vi "Autonomous.vi"   [LabVIEW 2017]
doc: "This VI starts when autonomous period begins, and will automatically be terminated when it ends. You can carry out timed or sensor driven operations directly to I/O or to subsystems without needing to return to the caller."
uses:
  <vilib>/Rock Robotics/WPI/SafetyOutput/WPI_SafetyOutputConfigMenu.ctl
  <vilib>/Rock Robotics/WPI/Utilities/WPI_GetSetVariantRefNum.vi
  <vilib>/Rock Robotics/Network Tables/NT Read String.vi
  <vilib>/Rock Robotics/WPI/RobotDrive/WPI_RobotDriveMecanumDrive_Cartesian.vi
types:
  T1 = typedef "WPI_JoystickDevRef.ctl" = cluster{"Device":T2}
  T2 = typedef "WPI_JoystickDeviceEnum.ctl" = enum16{"USB 0", "USB 1", "USB 2", "USB 3", "USB 4", "USB 5"}
  T3 = typedef "WPI_SafetyOutputConfigMenu.ctl" = enum16{"Enable", "Disable"}
  T4 = typedef "WPI_RobotDriveDevRef.ctl" = cluster{"DevStatus":errorcluster, "Motors[]":T5[], "Square Inputs":bool, "Max Output":dbl}
  T5 = typedef "WPI_MotorControlDeviceRef.ctl" = cluster{"DeviceStatus":errorcluster, "Type":T6, "PWM":cluster{"PWM Channel":T7, "DeadBand":T8}, "CAN":cluster{"Device Number":u8, "SetOutput VI Ref":variant, "GetOutput VI Ref":variant, "Enable VI Ref":variant, "Disable VI Ref":variant, "Data":variant}, "Invert":bool, "DIO PWM":cluster{"PWM \"Enable\" Channel":T7, "DIOChannel":T9, "PWM Rate":dbl}}
  T6 = typedef "WPI_MotorControlType.ctl" = enum16{"PWM", "CAN", "DIO PWM"}
  T7 = typedef "FPGA_DIOPWMChannel.ctl" = enum8{"PWM 0", "PWM 1", "PWM 2", "PWM 3", "PWM 4", "PWM 5", "PWM 6", "PWM 7", "PWM 8", "PWM 9", "PWM MXP 0", "PWM MXP 1", "PWM MXP 2", "PWM MXP 3", "PWM MXP 4", "PWM MXP 5", "PWM MXP 6", "PWM MXP 7", "PWM MXP 8", "PWM MXP 9", "Invalid"}
  T8 = typedef "WPI_PWMDeadband.ctl" = cluster{"Name":string, "maxPositivePwm":i32, "minPositivePwm":i32, "centerPwm":i32, "maxNegativePwm":i32, "minNegativePwm":i32, "angularRange":u16}
  T9 = typedef "FPGA_DIOChannel.ctl" = enum8{"DIO 0", "DIO 1", "DIO 2", "DIO 3", "DIO 4", "DIO 5", "DIO 6", "DIO 7", "DIO 8", "DIO 9", "DIO MXP 0", "DIO MXP 1", "DIO MXP 2", "DIO MXP 3", "DIO MXP 4", "DIO MXP 5", "DIO MXP 6", "DIO MXP 7", "DIO MXP 8", "DIO MXP 9", "DIO MXP 10", "DIO MXP 11", "DIO MXP 12", "DIO MXP 13", "DIO MXP 14", "DIO MXP 15", "SPI Port CS1", "SPI Port CS2", "SPI Port CS3", "SPI Port MISO", "SPI Port MOSI", "Invalid"}
  T10 = typedef "Command Status Info.ctl" = cluster{"Name":string, "Status":T11, "notifier out":T12}
  T11 = typedef "Completion Status.ctl" = enum16{"Successful", "Aborted", "Incomplete"}
  T12 = typedef "Completion Notifier.ctl" = refnum<notifier>
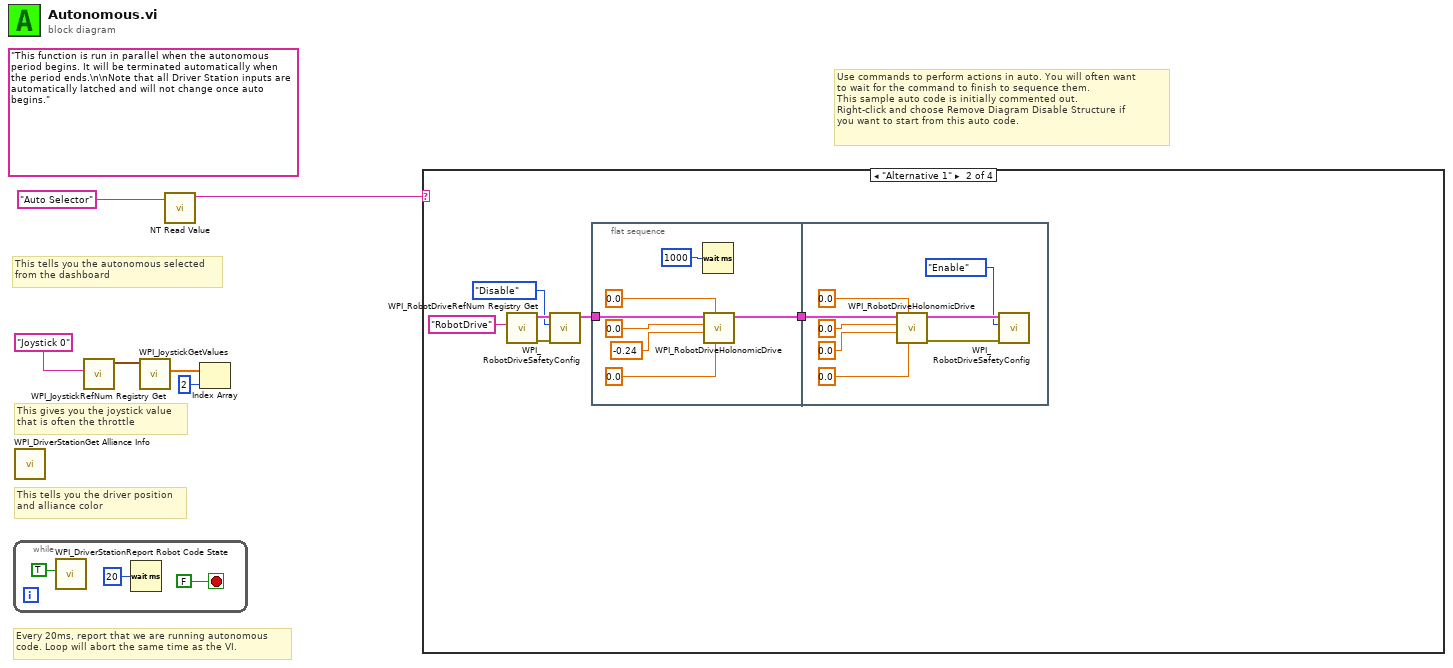
[diagram p0: block diagram]
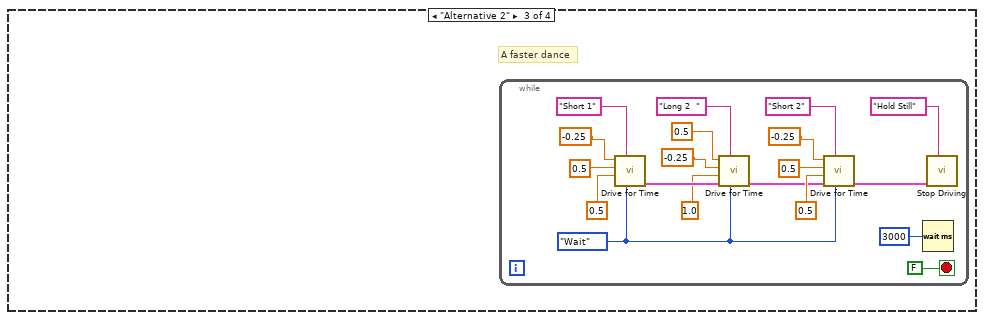
[diagram p3: hidden frame]
diagram:
  (unwired) "This function is run in parallel when the autonomous period begins. It will be terminated automatically when the period ends.\n\nNote that all Driver Station inputs are automatically latched and will not change once auto begins."
  # "This tells you the autonomous selected\nfrom the dashboard"
  # "Every 20ms, report that we are running autonomous\ncode. Loop will abort the same time as the VI."
  # "This gives you the joystick value\nthat is often the throttle"
  # "Use commands to perform actions in auto. You will often want\nto wait for the command to finish to sequence them.\nThis sample auto code is initially commented out. \nRight-click and choose Remove Diagram Disable Structure if\nyou want to start from this auto code."
  # "This tells you the driver position\nand alliance color"
  n1 = while {
    stop <- FALSE stop-if-true
    n2 = call <vilib>:"WPI_DriverStationReport Robot Code State.vi"("Autonomous"=TRUE) -> ()  [unwired: 10 in, 1 out]
    n3 = Wait (ms)(milliseconds to wait=u32 20) -> ()  [unwired: 1 out]
  }
  n4 = call <vilib>:"WPI_DriverStationGet Alliance Info.vi"() -> ()  [unwired: 12 out]
  n5 = call <vilib>:"WPI_JoystickRefNum Registry Get.vi"("refnum name"="Joystick 0") -> ("JoystickDevRef"=w5:T1)  [unwired: 1 in, 9 out]
  n6 = call <vilib>:"WPI_JoystickGetValues.vi"("JoystickDevRef"=w5) -> ("Axes"=w4:dbl[])  [unwired: 6 in, 4 out]
  n7 = call-poly <vilib>:"NT Read Value.vi"("Name"="Auto Selector") -> ("String"=w1:string)  [unwired: 9 in, 1 out]
  n8 = Index Array(array=w4, index=2) -> ()  [unwired: 1 out]
  n9 = case shown="\"Alternative 1\"" w1 {
    frame Default {
      # "You can put your main auto here, or you can right-click on the case and make any\nother frame be the default case."
      # "This is the frame that will execute if no selection is made, or if it is not recognized"
    }
    frame "Alternative 1" {
      n10 = call <vilib>:"WPI_RobotDriveRefNum Registry Get.vi"("refnum name"="RobotDrive") -> ("error out"=w13:errorcluster, "RobotDriveDevRef"=w14:T4)  [unwired: 9 in]
      n11 = call <vilib>:"WPI_RobotDriveSafetyConfig.vi"("error in (no error)"=w13, "mode"=WPI_SafetyOutputConfigMenu."Disable", "RobotDriveDevRef"=w14) -> ("RobotDriveDevRef"=w11:T4)  [unwired: 7 in, 1 out]
      n12 = flat-sequence {
        tunnel: w11 -> [w22]
        tunnel: [w16] -> w10
        tunnel: w10 -> [w30]
        frame #0 {
          n13 = Wait (ms)(milliseconds to wait=u32 1000) -> ()  [unwired: 1 out]
          n14 = call-poly <vilib>:"WPI_RobotDriveHolonomicDrive.vi"("Rotation"=0.0, "Gyro Angle"=0.0, "Y"=-0.24, "X"=0.0, "RobotDriveDevRef"=w22) -> ("RobotDriveDevRef"=w16:T4)  [unwired: 4 in, 2 out]
        }
        frame #1 {
          n15 = call-poly <vilib>:"WPI_RobotDriveHolonomicDrive.vi"("Rotation"=0.0, "Gyro Angle"=0.0, "Y"=0.0, "X"=0.0, "RobotDriveDevRef"=w30) -> ("error out"=w24:errorcluster, "RobotDriveDevRef"=w25:T4)  [unwired: 4 in, 1 out]
          n16 = call <vilib>:"WPI_RobotDriveSafetyConfig.vi"("error in (no error)"=w24, "mode"=WPI_SafetyOutputConfigMenu."Enable", "RobotDriveDevRef"=w25) -> ()  [unwired: 7 in, 2 out]
        }
      }
    }
    frame "Alternative 2" {
      # "A faster dance"
      n17 = while {
        stop <- FALSE stop-if-true
        w31 = enum16{"Start", "Wait"}."Wait" ("Synchronication")
        n18 = call "Drive for Time.vi"("Synchronization"=w31, "Description"="Short 1", "Seconds"=0.5 ("Delay (s)"), "Right Speed"=0.5 ("X axis value"), "Left Speed"=-0.25 ("X axis value")) -> ("Command Info Out"=w49:T10)  [unwired: 5 in, 1 out]
        n19 = call "Drive for Time.vi"("Synchronization"=w31, "Description"="Long 2  ", "Command Info In"=w49, "Seconds"=1.0 ("Delay (s)"), "Right Speed"=-0.25 ("X axis value"), "Left Speed"=0.5 ("X axis value")) -> ("Command Info Out"=w33:T10)  [unwired: 4 in, 1 out]
        n20 = call "Drive for Time.vi"("Synchronization"=w31, "Description"="Short 2", "Command Info In"=w33, "Seconds"=0.5 ("Delay (s)"), "Right Speed"=0.5 ("X axis value"), "Left Speed"=-0.25 ("X axis value")) -> ("Command Info Out"=w32:T10)  [unwired: 4 in, 1 out]
        n21 = Wait (ms)(milliseconds to wait=u32 3000 ("millisecond timer value")) -> ()  [unwired: 1 out]
        n22 = call "Stop Driving.vi"("Description"="Hold Still", "Command Info In"=w32) -> ()  [unwired: 9 in, 1 out]
      }
    }
    frame "Your Turn" {
    }
  }
